vi "Encode Base64.vi"(0 "normal string":string, 1 "line separator (\\n)":string="\n") -> (2 "base64 string":string)   [LabVIEW 2017, in "Encode Base64.lvlib"]
uses:
  Encode Base64.lvlib
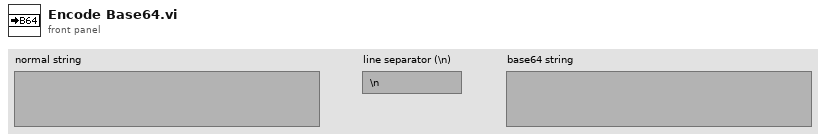
[diagram p1: front panel]
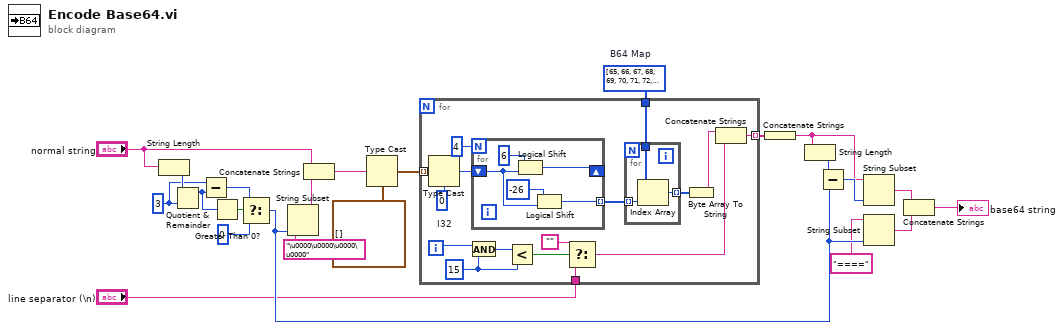
[diagram p0: block diagram]
diagram:
  w11 = u8[] [65, 66, 67, 68, 69, 70, 71, 72, 73, 74, 75, 76, 77, 78, 79, 80, 81, 82, 83, 84, 85, 86, 87, 88, 89, 90, 97, 98, 99, 100, 101, 102, 103, 104, 105, 106, 107, 108, 109, 110, 111, 112, 113, 114, 115, 116, 117, 118, 119, 120, 121, 122, 48, 49, 50, 51, 52, 53, 54, 55, 56, 57, 43, 47]  # B64 Map
  w17 = 3 ("y")
  n1 = String Length(string="normal string") -> (length=w18:i32)
  n2 = Quotient & Remainder(x=w18, y=w17) -> (x-y*floor(x/y)=w16:i32)  [unwired: 1 out]
  n3 = Subtract(x=w17, y=w16) -> (x-y=w13:i32)
  n4 = Greater Than 0?(x=w16) -> (x > 0?=w15:bool)
  n5 = Select(t=w13, s=w15, f=0 ("y")) -> (s? t:f=w8:i32)
  n6 = String Subset(string="\u0000\u0000\u0000\u0000", length (rest)=w8) -> (substring=w22:string)  [unwired: 1 out]
  n7 = Concatenate Strings("normal string", w22) -> (w20:string)
  n8 = Type Cast(type=cluster{"u8":u8, "u8":u8, "u8":u8}[] [], x=w20) -> (*(type *) &x=w12:cluster{"u8":u8, "u8":u8, "u8":u8}[])
  n9 = for {
    tunnel: w12 -> [w39] mode=indexing
    tunnel: w11 -> [w33]
    tunnel: "line separator (\\n)" -> [w26]
    tunnel: [w24] -> w2 mode=indexing
    i -> [w29]
    w30 = 15 ("x")
    w38 = 0  # I32
    n10 = Type Cast(type=w38, x=w39) -> (*(type *) &x=w37:i32)
    n11 = And(x=w29, y=w30) -> (x .and. y?=w31:i32)
    n12 = for {
      N: 4 -> [_]
      shift-right: [w47] -> _
      shift-left: w37 -> [w44]
      tunnel: [w43] -> w34 mode=indexing
      n13 = Logical Shift(y=6, x=w44) -> (x << y=w47:i32)
      n14 = Logical Shift(y=-26, x=w44) -> (x << y=w43:i32)
    }
    n15 = Less?(x=w31, y=w30) -> (x < y?=w28:bool)
    n16 = Select(t="", s=w28, f=w26) -> (s? t:f=w25:string)
    n17 = for {
      tunnel: w34 -> [w42] mode=indexing
      tunnel: w33 -> [w41]
      tunnel: [w40] -> w32 mode=indexing
      n18 = Index Array(array=w41, index=w42) -> (element=w40:u8)
    }
    n19 = Byte Array To String(unsigned byte array=w32) -> (string=w36:string)
    n20 = Concatenate Strings(w36, w25) -> (w24:string)
  }
  n21 = Concatenate Strings(w2) -> (w1:string)
  n22 = String Length(string=w1) -> (length=w10:i32)
  n23 = Subtract(x=w10, y=w8) -> (x-y=w9:i32)
  n24 = String Subset(string=w1, length (rest)=w9) -> (substring=w6:string)  [unwired: 1 out]
  n25 = String Subset(string="====", length (rest)=w8) -> (substring=w5:string)  [unwired: 1 out]
  n26 = Concatenate Strings(w6, w5) -> (→"base64 string":string)
